vi "Run Bfr Rx - Cached - Check Cache.vi"(7 "Cache Size":u64, 8 "error in (no error)":errorcluster, 10 "Data in":u8[](array[numeric]), 11 "Data Offset in":u64) -> (0 "error out":errorcluster, 2 "Data out":u8[](array[numeric]), 4 "Copy and Flush":bool, 6 "Data Size out":u64)   [LabVIEW 2019, in "UDP-Custom-Device Engine.lvlib"]
uses:
  UDP-Custom-Device Engine.lvlib
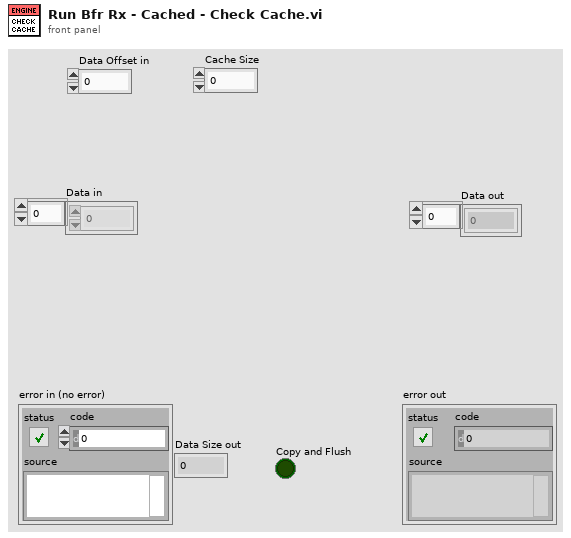
[diagram p1: front panel]
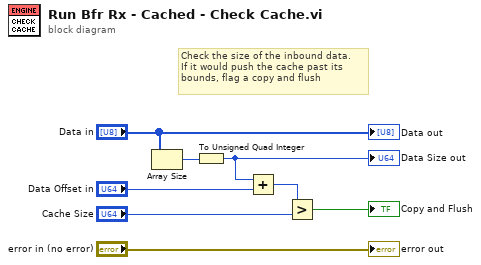
[diagram p0: block diagram]
diagram:
  # "Check the size of the inbound data.\nIf it would push the cache past its\nbounds, flag a copy and flush"
  n1 = Array Size(array="Data in") -> (size(s)=w3:i32)
  n2 = To Unsigned Quad Integer(1:w3) -> (0:w2:u64)
  "Data Size out" <- w2
  n3 = Add(x=w2, y="Data Offset in") -> (x+y=w5:u64)
  n4 = Greater?(x=w5, y="Cache Size") -> (0:→"Copy and Flush":bool)
  "error out" <- "error in (no error)"
  "Data out" <- "Data in"
